vi "Read Connection ID.vi"(8 "error in (no error)":errorcluster, 11 "RawSocket Handler in":refnum<class "RawSocket TCP Handler.lvclass">) -> (0 "error out":errorcluster, 2 "Connection ID":refnum<k5>, 3 "RawSocket Handler out":refnum<class "RawSocket TCP Handler.lvclass">)   [LabVIEW 2021, in "wamplv.lvlib" / "RawSocket TCP Handler.lvclass"]
uses:
  RawSocket TCP Handler.lvclass
  RawSocket TCP Handler.lvclass/RawSocket TCP Handler.ctl
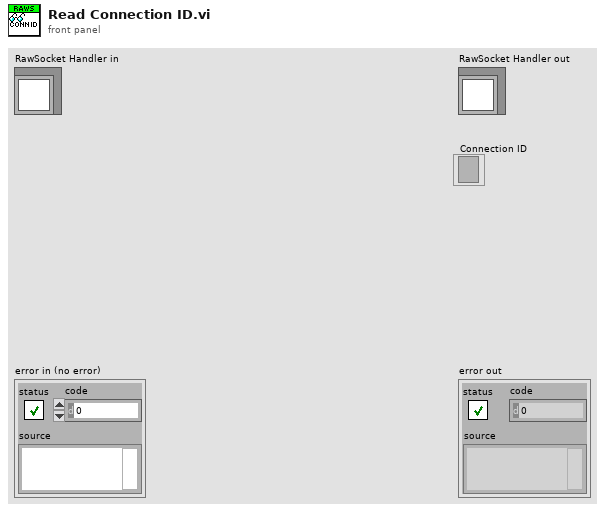
[diagram p1: front panel]
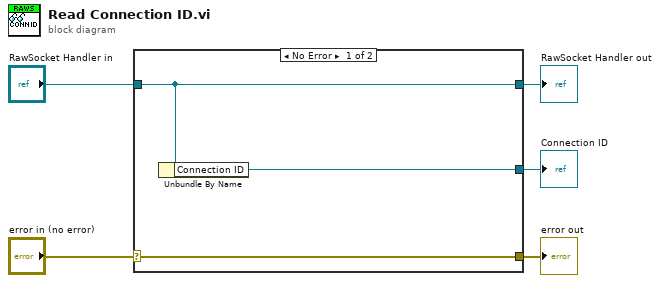
[diagram p0: block diagram]
diagram:
  n1 = case shown="No Error" "error in (no error)" {
    selector: "error in (no error)" -> [w8 w9]
    tunnel: [w8 w9] -> w4
    tunnel: [w7 w10] -> w2
    tunnel: "RawSocket Handler in" -> [w7 w10]
    tunnel: [w6 _] -> w1
    frame No Error {
      n2 = Unbundle By Name(w7) -> ("Connection ID"=w6:refnum<k5>)
    }
    frame Error {
    }
  }
  "error out" <- w4
  "RawSocket Handler out" <- w2
  "Connection ID" <- w1
